vi "niRFUtil RFHS Channelizer CreateChannelizerCheck CSG.vi"(0 "Channel Spec":T1={"freq in Hz"=TRUE, "Filter Type Hint"=enum."FFT (LTE)", "Hint Value"=0.5, "Channels"=[]} {"Channels"."Flags" items=["None"=0, "Force Fractional"=1, "Use Multistage"=2, "Use Pretrigger Data "=256, "Frequency Shift Only"=4]; "Channels"."fs" format="%#_8p"; "Channels"."fc" format="%#_6p"; "Channels"."stopBW" format="%#_6p"; "Channels"."passBW" format="%#_6p"; "Hint Value" format="%#_8p"}, 5 "fs [Hz]":dbl=1000000000.0 format="%#_6p", 11 "error in (no error)":errorcluster) -> (4 "Channel Spec (out)":T1={"freq in Hz"=TRUE, "Filter Type Hint"=enum."Auto", "Hint Value"=0.0, "Channels"=[]} {"Channels"."Flags" items=["None"=0, "Force Fractional"=1, "Use Multistage"=2, "Use Pretrigger Data "=256, "Frequency Shift Only"=4]; "Channels"."fs" format="%#_8p"; "Channels"."fc" format="%#_6p"; "Channels"."stopBW" format="%#_6p"; "Channels"."passBW" format="%#_6p"; "Hint Value" format="%#_8p"}, 15 "error out":errorcluster)   [LabVIEW 2015, in "niRFUtil.lvlib"]
uses:
  niRFUtil.lvlib
  Includes/niRFUtil RFHS Channelizer ChannelSpecification.ctl
  Includes/niRFUtil RFHS Channelizer FilterTypeHint.ctl
  Includes/niRFUtil RFHS Channelizer ChannelSpecificationBase.ctl
  Includes/niRFUtil RFHS Channelizer ChannelFlags.ctl
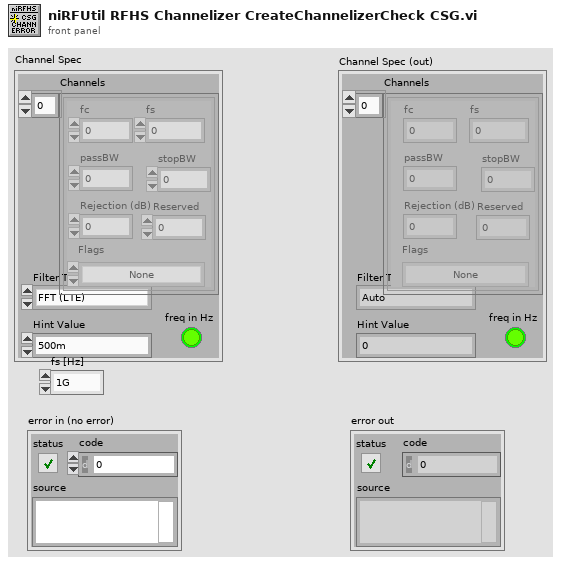
[diagram p1: front panel]
types:
  T1 = typedef "niRFUtil.lvlib/niRFUtil RFHS Channelizer ChannelSpecification.ctl" = cluster{"freq in Hz":bool, "Filter Type Hint":T2, "Hint Value":dbl, "Channels":T3[]}
  T2 = typedef "niRFUtil.lvlib/niRFUtil RFHS Channelizer FilterTypeHint.ctl" = enum16{"Auto", "FFT (LTE)", "FFT (WiFi)", "FFT (custom)"}
  T3 = typedef "niRFUtil.lvlib/niRFUtil RFHS Channelizer ChannelSpecificationBase.ctl" = cluster{"fc":dbl, "fs":dbl, "passBW":dbl, "stopBW":dbl, "Rejection (dB)":dbl, "Flags":T4, "Reserved":i32}
  T4 = typedef "niRFUtil.lvlib/niRFUtil RFHS Channelizer ChannelFlags.ctl" = u32
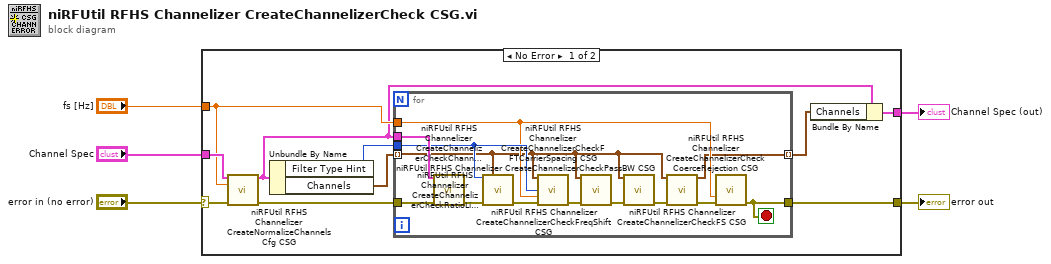
[diagram p0: block diagram]
diagram:
  n1 = case shown="No Error" "error in (no error)" {
    selector: "error in (no error)" -> [w8 w29]
    tunnel: "fs [Hz]" -> [w9 _]
    tunnel: [w15 w29] -> w4
    tunnel: "Channel Spec" -> [w10 _]
    tunnel: [w13 _] -> w2
    frame No Error {
      n2 = call "niRFUtil RFHS Channelizer CreateNormalizeChannelsCfg CSG.vi"("Channel Spec"=w10, "fs [Hz]"=w9, "error in (no error)"=w8) -> ("Channel Spec (out)"=w6:T1, "error out"=w7:errorcluster)  [unwired: 11 in]
      n3 = Unbundle By Name(w6) -> ("Filter Type Hint"=w12:T2, "Channels"=w11:T3[])
      n4 = for {
        tunnel: w6 -> [w21]
        tunnel: w7 -> [w22]
        tunnel: w9 -> [w19]
        tunnel: [w16] -> w15
        tunnel: w11 -> [w17] mode=indexing
        tunnel: [w18] -> w14 mode=indexing
        tunnel: w12 -> [w20]
        stop <- w16 stop-if-true
        n5 = call "niRFUtil RFHS Channelizer CreateChannelizerCheckChannelNum CSG.vi"("Channel Spec"=w21, "error in (no error)"=w22) -> ("error out"=w23:errorcluster)  [unwired: 13 in]
        n6 = call "niRFUtil RFHS Channelizer CreateChannelizerCheckRatioLimits CSG.vi"("Filter Type Hint"=w20, "Channel Spec Base in"=w17, "error in (no error)"=w23) -> ("error out"=w24:errorcluster)  [unwired: 12 in]
        n7 = call "niRFUtil RFHS Channelizer CreateChannelizerCheckFFTCarrierSpacing CSG.vi"("Channel Spec Base in"=w17, "Filter Type Hint"=w20, "fs [Hz]"=w19, "error in (no error)"=w24) -> ("error out"=w25:errorcluster)  [unwired: 11 in]
        n8 = call "niRFUtil RFHS Channelizer CreateChannelizerCheckFreqShift CSG.vi"("Channel Spec Base in"=w17, "error in (no error)"=w25) -> ("error out"=w26:errorcluster)  [unwired: 13 in]
        n9 = call "niRFUtil RFHS Channelizer CreateChannelizerCheckPassBW CSG.vi"("Channel Spec Base in"=w17, "error in (no error)"=w26) -> ("error out"=w27:errorcluster)  [unwired: 13 in]
        n10 = call "niRFUtil RFHS Channelizer CreateChannelizerCheckCoerceRejection CSG.vi"("Channel Spec Base in"=w17, "error in (no error)"=w27) -> ("Channel Spec Base out"=w18:T3, "error out"=w28:errorcluster)  [unwired: 12 in]
        n11 = call "niRFUtil RFHS Channelizer CreateChannelizerCheckFS CSG.vi"("fs [Hz]"=w19, "error in (no error)"=w28) -> ("error out"=w16:errorcluster)  [unwired: 13 in]
      }
      n12 = Bundle By Name(cluster=w6, "Channels"=w14) -> (w13:T1)
    }
    frame Error {
    }
  }
  "error out" <- w4
  "Channel Spec (out)" <- w2
